vi "Isomap.vi"(8 "error in":errorcluster) -> (0 "error out":errorcluster, 3 "out":refnum<class "Isomap.lvclass">)   [LabVIEW 2020]
doc: "Isomap Embedding\n\n Non-linear dimensionality reduction through Isometric Mapping\n\n Read more in the :ref:`User Guide <isomap>`.\n\n Parameters\n ----------\n n_neighbors : int, default=5\n number of neighbors to consider for each point.\n\n n_components : int, default=2\n number of coordinates for the manifold\n\n eigen_solver : {'auto', 'arpack', 'dense'}, default='auto'\n 'auto' : Attempt to choose the most efficient solver\n for the given problem.\n\n 'arpack' : Use Arnoldi decomposition to find the eigenvalues\n and eigenvectors.\n\n 'dense' : Use a direct solver (i.e. LAPACK)\n for the eigenvalue decomposition.\n\n tol : float, default=0\n Convergence tolerance passed to arpack or lobpcg.\n not used if eigen_solver == 'dense'.\n\n max_iter : int, default=None\n Maximum number of iterations for the arpack solver.\n not used if eigen_solver == 'dense'.\n\n path_method : {'auto', 'FW', 'D'}, default='auto'\n Method to use in finding shortest path.\n\n 'auto' : attempt to choose the best algorithm automatically.\n\n 'FW' : Floyd-Warshall algorithm.\n\n 'D' : Dijkstra's algorithm.\n\n neighbors_algorithm : {'auto', 'brute', 'kd_tree', 'ball_tree'}, default='auto'\n Algorithm to use for nearest neighbors search,\n passed to neighbors.NearestNeighbors instance.\n\n n_jobs : int or None, default=None\n The number of parallel jobs to run.\n ``None`` means 1 unless in a :obj:`joblib.parallel_backend` context.\n ``-1`` means using all processors. See :term:`Glossary <n_jobs>`\n for more details.\n\n metric : string, or callable, default=\"minkowski\"\n The metric to use when calculating distance between instances in a\n feature array. If metric is a string or callable, it must be one of\n the options allowed by :func:`sklearn.metrics.pairwise_distances` for\n its metric parameter.\n If metric is \"precomputed\", X is assumed to be a distance matrix and\n must be square. X may be a :term:`Glossary <sparse graph>`.\n\n .. versionadded:: 0.22\n\n p : int, default=2\n Parameter for the Minkowski metric from\n sklearn.metrics.pairwise.pairwise_distances. When p = 1, this is\n equivalent to using manhattan_distance (l1), and euclidean_distance\n (l2) for p = 2. For arbitrary p, minkowski_distance (l_p) is used.\n\n .. versionadded:: 0.22\n\n metric_params : dict, default=None\n Additional keyword arguments for the metric function.\n\n .. versionadded:: 0.22\n\n Attributes\n ----------\n embedding_ : array-like, shape (n_samples, n_components)\n Stores the embedding vectors.\n\n kernel_pca_ : object\n :class:`~sklearn.decomposition.KernelPCA` object used to implement the\n embedding.\n\n nbrs_ : sklearn.neighbors.NearestNeighbors instance\n Stores nearest neighbors instance, including BallTree or KDtree\n if applicable.\n\n dist_matrix_ : array-like, shape (n_samples, n_samples)\n Stores the geodesic distance matrix of training data.\n\n \nAvailable methods:\nFit\nFit Transform\nGet Attributes\nGet Params\nSet Params"
uses:
  Isomap.lvclass
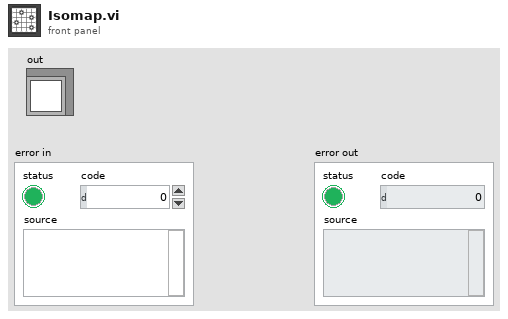
[diagram p1: front panel]
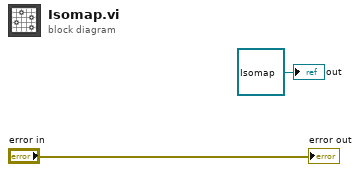
[diagram p0: block diagram]
diagram:
  "out" <- refnum<class "Isomap.lvclass"> refnum ("model")
  "error out" <- "error in"
